vi "Scripted Autonmous V1.vi"(9 "All Autonmous Programs":T32, 10 "Autonmous Program":T1, 11 "Robot dev revs":T3={"Drive"={"Drive Actuaters"={"Motor devRevs"={"Left Side Motors"={"Motor 1 devRev"={"DeviceStatus"={"status"=FALSE, "code"=0, "source"=""}, "Type"=enum."PWM", "PWM"={"Digital Module"=enum."Digital Module 1", "PWM Channel"=enum."PWM 1", "DeadBand"={"Name"="", "maxPositivePwm"=0, "minPositivePwm"=0, "centerPwm"=0, "maxNegativePwm"=0, "minNegativePwm"=0, "angularRange"=0}}, "CAN"={"Device Number"=0, "Control Mode"=enum."Percent VBus", "Semaphore"=refnum, "Max Vout"=0.0}, "Invert"=FALSE, "TransformRef"=refnum, "InvTransformRef"=refnum}, "Motor 2 devRev"={"DeviceStatus"={"status"=FALSE, "code"=0, "source"=""}, "Type"=enum."PWM", "PWM"={"Digital Module"=enum."Digital Module 1", "PWM Channel"=enum."PWM 1", "DeadBand"={"Name"="", "maxPositivePwm"=0, "minPositivePwm"=0, "centerPwm"=0, "maxNegativePwm"=0, "minNegativePwm"=0, "angularRange"=0}}, "CAN"={"Device Number"=0, "Control Mode"=enum."Percent VBus", "Semaphore"=refnum, "Max Vout"=0.0}, "Invert"=FALSE, "TransformRef"=refnum, "InvTransformRef"=refnum}, "Motor 3 devRev"={"DeviceStatus"={"status"=FALSE, "code"=0, "source"=""}, "Type"=enum."PWM", "PWM"={"Digital Module"=enum."Digital Module 1", "PWM Channel"=enum."PWM 1", "DeadBand"={"Name"="", "maxPositivePwm"=0, "minPositivePwm"=0, "centerPwm"=0, "maxNegativePwm"=0, "minNegativePwm"=0, "angularRange"=0}}, "CAN"={"Device Number"=0, "Control Mode"=enum."Percent VBus", "Semaphore"=refnum, "Max Vout"=0.0}, "Invert"=FALSE, "TransformRef"=refnum, "InvTransformRef"=refnum}}, "Right Side Motors"={"Motor 1 devRev"={"DeviceStatus"={"status"=FALSE, "code"=0, "source"=""}, "Type"=enum."PWM", "PWM"={"Digital Module"=enum."Digital Module 1", "PWM Channel"=enum."PWM 1", "DeadBand"={"Name"="", "maxPositivePwm"=0, "minPositivePwm"=0, "centerPwm"=0, "maxNegativePwm"=0, "minNegativePwm"=0, "angularRange"=0}}, "CAN"={"Device Number"=0, "Control Mode"=enum."Percent VBus", "Semaphore"=refnum, "Max Vout"=0.0}, "Invert"=FALSE, "TransformRef"=refnum, "InvTransformRef"=refnum}, "Motor 2 devRev"={"DeviceStatus"={"status"=FALSE, "code"=0, "source"=""}, "Type"=enum."PWM", "PWM"={"Digital Module"=enum."Digital Module 1", "PWM Channel"=enum."PWM 1", "DeadBand"={"Name"="", "maxPositivePwm"=0, "minPositivePwm"=0, "centerPwm"=0, "maxNegativePwm"=0, "minNegativePwm"=0, "angularRange"=0}}, "CAN"={"Device Number"=0, "Control Mode"=enum."Percent VBus", "Semaphore"=refnum, "Max Vout"=0.0}, "Invert"=FALSE, "TransformRef"=refnum, "InvTransformRef"=refnum}, "Motor 3 devRev"={"DeviceStatus"={"status"=FALSE, "code"=0, "source"=""}, "Type"=enum."PWM", "PWM"={"Digital Module"=enum."Digital Module 1", "PWM Channel"=enum."PWM 1", "DeadBand"={"Name"="", "maxPositivePwm"=0, "minPositivePwm"=0, "centerPwm"=0, "maxNegativePwm"=0, "minNegativePwm"=0, "angularRange"=0}}, "CAN"={"Device Number"=0, "Control Mode"=enum."Percent VBus", "Semaphore"=refnum, "Max Vout"=0.0}, "Invert"=FALSE, "TransformRef"=refnum, "InvTransformRef"=refnum}}, "dev Status"={"status"=FALSE, "code"=0, "source"=""}}, "SolenoidDevRef"={"DevStatus"={"status"=FALSE, "code"=0, "source"=""}, "Solenoid Module"=enum."Solenoid Module 1", "Forward Solenoid Channel"=enum."Solenoid 1", "Reverse Solenoid Channel"=enum."Solenoid 1"}}, "Drive Sensor data"={"Encoders"={"Right Encoder"={"DevStatus"={"status"=FALSE, "code"=0, "source"=""}, "EncoderIndex"=enum."Enc 0", "CounterIndex"=enum."Ctr 0", "DistancePerCount"=0.0, "Decoding Type"=enum."1x"}}, "GyroDevRef"={"DevStatus"={"status"=FALSE, "code"=0, "source"=""}, "Analog Module"=enum."Analog Module 1", "Analog Channel"=enum."AI 1", "Offset"=0.0, "Gain (VoltsPerDegree/Second)"=0.0}, "Last commanded Angle"=0.0}}, "Catapult devrevs"={"MotorControlDeviceRef"={"DeviceStatus"={"status"=FALSE, "code"=0, "source"=""}, "Type"=enum."PWM", "PWM"={"Digital Module"=enum."Digital Module 1", "PWM Channel"=enum."PWM 1", "DeadBand"={"Name"="", "maxPositivePwm"=0, "minPositivePwm"=0, "centerPwm"=0, "maxNegativePwm"=0, "minNegativePwm"=0, "angularRange"=0}}, "CAN"={"Device Number"=0, "Control Mode"=enum."Percent VBus", "Semaphore"=refnum, "Max Vout"=0.0}, "Invert"=FALSE, "TransformRef"=refnum, "InvTransformRef"=refnum}, "SolenoidDevRef"={"DevStatus"={"status"=FALSE, "code"=0, "source"=""}, "Solenoid Module"=enum."Solenoid Module 1", "Forward Solenoid Channel"=enum."Solenoid 1", "Reverse Solenoid Channel"=enum."Solenoid 1"}, "first limit switch"={"DevStatus"={"status"=FALSE, "code"=0, "source"=""}, "DIO Channel"=enum."DIO 1", "Digital Module"=enum."Digital Module 1"}, "second limit switch"={"DevStatus"={"status"=FALSE, "code"=0, "source"=""}, "DIO Channel"=enum."DIO 1", "Digital Module"=enum."Digital Module 1"}}, "Drive Joystick"={"Device"=enum."USB 1"}, "Operator Joystick"={"Device"=enum."USB 1"}, "roller devrevs"={"SolenoidDevRef"={"DevStatus"={"status"=FALSE, "code"=0, "source"=""}, "Solenoid Module"=enum."Solenoid Module 1", "Forward Solenoid Channel"=enum."Solenoid 1", "Reverse Solenoid Channel"=enum."Solenoid 1"}, "MotorControlDeviceRef"={"DeviceStatus"={"status"=FALSE, "code"=0, "source"=""}, "Type"=enum."PWM", "PWM"={"Digital Module"=enum."Digital Module 1", "PWM Channel"=enum."PWM 1", "DeadBand"={"Name"="", "maxPositivePwm"=0, "minPositivePwm"=0, "centerPwm"=0, "maxNegativePwm"=0, "minNegativePwm"=0, "angularRange"=0}}, "CAN"={"Device Number"=0, "Control Mode"=enum."Percent VBus", "Semaphore"=refnum, "Max Vout"=0.0}, "Invert"=FALSE, "TransformRef"=refnum, "InvTransformRef"=refnum}, "DigitalInputDevRef"={"DevStatus"={"status"=FALSE, "code"=0, "source"=""}, "DIO Channel"=enum."Invalid", "Digital Module"=enum."Digital Module 1"}}, "Puncher devrevs"={"SolenoidDevRef"={"DevStatus"={"status"=FALSE, "code"=0, "source"=""}, "Solenoid Module"=enum."Solenoid Module 1", "Forward Solenoid Channel"=enum."Solenoid 1", "Reverse Solenoid Channel"=enum."Solenoid 1"}, "DigitalInputDevRef"={"DevStatus"={"status"=FALSE, "code"=0, "source"=""}, "DIO Channel"=enum."DIO 1", "Digital Module"=enum."Digital Module 1"}}}) -> (3 "Robot dev revs out":T3={"Drive"={"Drive Actuaters"={"Motor devRevs"={"Left Side Motors"={"Motor 1 devRev"={"DeviceStatus"={"status"=FALSE, "code"=0, "source"=""}, "Type"=enum."PWM", "PWM"={"Digital Module"=enum."Digital Module 1", "PWM Channel"=enum."PWM 1", "DeadBand"={"Name"="", "maxPositivePwm"=0, "minPositivePwm"=0, "centerPwm"=0, "maxNegativePwm"=0, "minNegativePwm"=0, "angularRange"=0}}, "CAN"={"Device Number"=0, "Control Mode"=enum."Percent VBus", "Semaphore"=refnum, "Max Vout"=0.0}, "Invert"=FALSE, "TransformRef"=refnum, "InvTransformRef"=refnum}, "Motor 2 devRev"={"DeviceStatus"={"status"=FALSE, "code"=0, "source"=""}, "Type"=enum."PWM", "PWM"={"Digital Module"=enum."Digital Module 1", "PWM Channel"=enum."PWM 1", "DeadBand"={"Name"="", "maxPositivePwm"=0, "minPositivePwm"=0, "centerPwm"=0, "maxNegativePwm"=0, "minNegativePwm"=0, "angularRange"=0}}, "CAN"={"Device Number"=0, "Control Mode"=enum."Percent VBus", "Semaphore"=refnum, "Max Vout"=0.0}, "Invert"=FALSE, "TransformRef"=refnum, "InvTransformRef"=refnum}, "Motor 3 devRev"={"DeviceStatus"={"status"=FALSE, "code"=0, "source"=""}, "Type"=enum."PWM", "PWM"={"Digital Module"=enum."Digital Module 1", "PWM Channel"=enum."PWM 1", "DeadBand"={"Name"="", "maxPositivePwm"=0, "minPositivePwm"=0, "centerPwm"=0, "maxNegativePwm"=0, "minNegativePwm"=0, "angularRange"=0}}, "CAN"={"Device Number"=0, "Control Mode"=enum."Percent VBus", "Semaphore"=refnum, "Max Vout"=0.0}, "Invert"=FALSE, "TransformRef"=refnum, "InvTransformRef"=refnum}}, "Right Side Motors"={"Motor 1 devRev"={"DeviceStatus"={"status"=FALSE, "code"=0, "source"=""}, "Type"=enum."PWM", "PWM"={"Digital Module"=enum."Digital Module 1", "PWM Channel"=enum."PWM 1", "DeadBand"={"Name"="", "maxPositivePwm"=0, "minPositivePwm"=0, "centerPwm"=0, "maxNegativePwm"=0, "minNegativePwm"=0, "angularRange"=0}}, "CAN"={"Device Number"=0, "Control Mode"=enum."Percent VBus", "Semaphore"=refnum, "Max Vout"=0.0}, "Invert"=FALSE, "TransformRef"=refnum, "InvTransformRef"=refnum}, "Motor 2 devRev"={"DeviceStatus"={"status"=FALSE, "code"=0, "source"=""}, "Type"=enum."PWM", "PWM"={"Digital Module"=enum."Digital Module 1", "PWM Channel"=enum."PWM 1", "DeadBand"={"Name"="", "maxPositivePwm"=0, "minPositivePwm"=0, "centerPwm"=0, "maxNegativePwm"=0, "minNegativePwm"=0, "angularRange"=0}}, "CAN"={"Device Number"=0, "Control Mode"=enum."Percent VBus", "Semaphore"=refnum, "Max Vout"=0.0}, "Invert"=FALSE, "TransformRef"=refnum, "InvTransformRef"=refnum}, "Motor 3 devRev"={"DeviceStatus"={"status"=FALSE, "code"=0, "source"=""}, "Type"=enum."PWM", "PWM"={"Digital Module"=enum."Digital Module 1", "PWM Channel"=enum."PWM 1", "DeadBand"={"Name"="", "maxPositivePwm"=0, "minPositivePwm"=0, "centerPwm"=0, "maxNegativePwm"=0, "minNegativePwm"=0, "angularRange"=0}}, "CAN"={"Device Number"=0, "Control Mode"=enum."Percent VBus", "Semaphore"=refnum, "Max Vout"=0.0}, "Invert"=FALSE, "TransformRef"=refnum, "InvTransformRef"=refnum}}, "dev Status"={"status"=FALSE, "code"=0, "source"=""}}, "SolenoidDevRef"={"DevStatus"={"status"=FALSE, "code"=0, "source"=""}, "Solenoid Module"=enum."Solenoid Module 1", "Forward Solenoid Channel"=enum."Solenoid 1", "Reverse Solenoid Channel"=enum."Solenoid 1"}}, "Drive Sensor data"={"Encoders"={"Right Encoder"={"DevStatus"={"status"=FALSE, "code"=0, "source"=""}, "EncoderIndex"=enum."Enc 0", "CounterIndex"=enum."Ctr 0", "DistancePerCount"=0.0, "Decoding Type"=enum."1x"}}, "GyroDevRef"={"DevStatus"={"status"=FALSE, "code"=0, "source"=""}, "Analog Module"=enum."Analog Module 1", "Analog Channel"=enum."AI 1", "Offset"=0.0, "Gain (VoltsPerDegree/Second)"=0.0}, "Last commanded Angle"=0.0}}, "Catapult devrevs"={"MotorControlDeviceRef"={"DeviceStatus"={"status"=FALSE, "code"=0, "source"=""}, "Type"=enum."PWM", "PWM"={"Digital Module"=enum."Digital Module 1", "PWM Channel"=enum."PWM 1", "DeadBand"={"Name"="", "maxPositivePwm"=0, "minPositivePwm"=0, "centerPwm"=0, "maxNegativePwm"=0, "minNegativePwm"=0, "angularRange"=0}}, "CAN"={"Device Number"=0, "Control Mode"=enum."Percent VBus", "Semaphore"=refnum, "Max Vout"=0.0}, "Invert"=FALSE, "TransformRef"=refnum, "InvTransformRef"=refnum}, "SolenoidDevRef"={"DevStatus"={"status"=FALSE, "code"=0, "source"=""}, "Solenoid Module"=enum."Solenoid Module 1", "Forward Solenoid Channel"=enum."Solenoid 1", "Reverse Solenoid Channel"=enum."Solenoid 1"}, "first limit switch"={"DevStatus"={"status"=FALSE, "code"=0, "source"=""}, "DIO Channel"=enum."DIO 1", "Digital Module"=enum."Digital Module 1"}, "second limit switch"={"DevStatus"={"status"=FALSE, "code"=0, "source"=""}, "DIO Channel"=enum."DIO 1", "Digital Module"=enum."Digital Module 1"}}, "Drive Joystick"={"Device"=enum."USB 1"}, "Operator Joystick"={"Device"=enum."USB 1"}, "roller devrevs"={"SolenoidDevRef"={"DevStatus"={"status"=FALSE, "code"=0, "source"=""}, "Solenoid Module"=enum."Solenoid Module 1", "Forward Solenoid Channel"=enum."Solenoid 1", "Reverse Solenoid Channel"=enum."Solenoid 1"}, "MotorControlDeviceRef"={"DeviceStatus"={"status"=FALSE, "code"=0, "source"=""}, "Type"=enum."PWM", "PWM"={"Digital Module"=enum."Digital Module 1", "PWM Channel"=enum."PWM 1", "DeadBand"={"Name"="", "maxPositivePwm"=0, "minPositivePwm"=0, "centerPwm"=0, "maxNegativePwm"=0, "minNegativePwm"=0, "angularRange"=0}}, "CAN"={"Device Number"=0, "Control Mode"=enum."Percent VBus", "Semaphore"=refnum, "Max Vout"=0.0}, "Invert"=FALSE, "TransformRef"=refnum, "InvTransformRef"=refnum}, "DigitalInputDevRef"={"DevStatus"={"status"=FALSE, "code"=0, "source"=""}, "DIO Channel"=enum."Invalid", "Digital Module"=enum."Digital Module 1"}}, "Puncher devrevs"={"SolenoidDevRef"={"DevStatus"={"status"=FALSE, "code"=0, "source"=""}, "Solenoid Module"=enum."Solenoid Module 1", "Forward Solenoid Channel"=enum."Solenoid 1", "Reverse Solenoid Channel"=enum."Solenoid 1"}, "DigitalInputDevRef"={"DevStatus"={"status"=FALSE, "code"=0, "source"=""}, "DIO Channel"=enum."DIO 1", "Digital Module"=enum."Digital Module 1"}}})   [LabVIEW 2013]
uses:
  Auto Text file code/All Autonmous Programs typedef.ctl
  Auto Text file code/Autonmous Program typedef.ctl
  Auto Text file code/Autonmous Scripting array typedef.ctl
  Robot dev revs.ctl
  Drive Code/Drive typedef.ctl
  Drive Code/Drive Motors Typedef.ctl
  Drive Code/GearBox Typedef.ctl
  <vilib>/Rock Robotics/WPI/MotorControl/WPI_MotorControlDeviceRef.ctl
  <vilib>/Rock Robotics/SystemInterfaces/Typedef/FPGA_TypedefDigitalModule.ctl
  <vilib>/Rock Robotics/SystemInterfaces/DIO/FPGA_DIOPWMChannel.ctl
  <vilib>/Rock Robotics/WPI/PWM/WPI_PWMDeadband.ctl
  <vilib>/Rock Robotics/WPI/CAN/Jaguar/SubVIs/WPI_CANJaguar_ControlMode.ctl
  <vilib>/Rock Robotics/WPI/PWM/WPI_PWMTransform_ConPane.ctl
  <vilib>/Rock Robotics/WPI/Solenoid/WPI_SolenoidDevRef.ctl
  <vilib>/Rock Robotics/SystemInterfaces/Typedef/FPGA_TypedefSolenoidModule.ctl
  <vilib>/Rock Robotics/WPI/Solenoid/WPI_SolenoidChannel.ctl
  Drive Code/Drive Sensor Typedef.ctl
  <vilib>/Rock Robotics/WPI/Encoder/WPI_EncoderDevRef.ctl
  <vilib>/Rock Robotics/SystemInterfaces/Encoder/FPGA_EncoderIdx.ctl
  <vilib>/Rock Robotics/SystemInterfaces/Counter/FPGA_CounterCtrSystemIndex.ctl
  <vilib>/Rock Robotics/WPI/Encoder/WPI_EncoderType.ctl
  <vilib>/Rock Robotics/WPI/Gyro/WPI_GyroDevRef.ctl
  <vilib>/Rock Robotics/SystemInterfaces/Typedef/FPGA_TypedefAnalogModule.ctl
  <vilib>/Rock Robotics/SystemInterfaces/AI/FPGA_AIChannel.ctl
  catapult code/catapult type def.ctl
  <vilib>/Rock Robotics/WPI/DigitalInput/WPI_DigitalInputDevRef.ctl
  <vilib>/Rock Robotics/SystemInterfaces/DIO/FPGA_DIOChannel.ctl
  <vilib>/Rock Robotics/WPI/Joystick/WPI_JoystickDevRef.ctl
  <vilib>/Rock Robotics/WPI/Joystick/WPI_JoystickDeviceEnum.ctl
  Roller V2/roller typedef.ctl
  Puncher/Puncher type.ctl
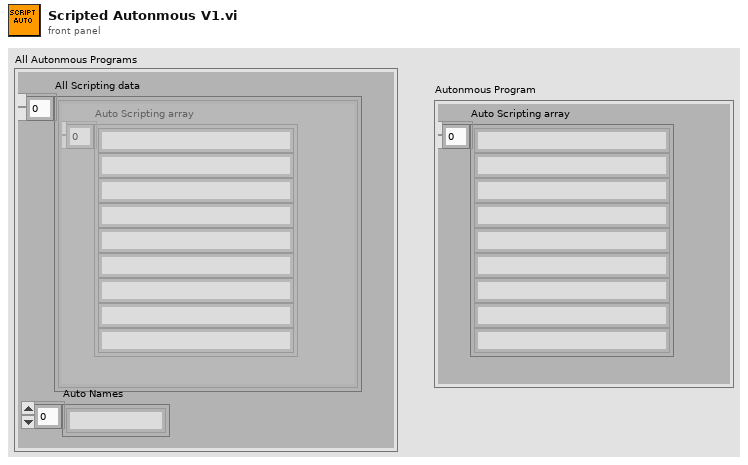
[diagram p1: front panel]
types:
  T1 = typedef "Autonmous Program typedef.ctl" = cluster{"Auto Scripting array":T2}
  T2 = typedef "Autonmous Scripting array typedef.ctl" = string[]
  T3 = typedef "Robot dev revs.ctl" = cluster{"Drive":T4, "Catapult devrevs":T25, "Drive Joystick":T28, "Operator Joystick":T28, "roller devrevs":T30, "Puncher devrevs":T31}
  T4 = typedef "Drive typedef.ctl" = cluster{"Drive Actuaters":cluster{"Motor devRevs":T5, "SolenoidDevRef":T14}, "Drive Sensor data":T17}
  T5 = typedef "Drive Motors Typedef.ctl" = cluster{"Left Side Motors":T6, "Right Side Motors":T6, "dev Status":errorcluster}
  T6 = typedef "GearBox Typedef.ctl" = cluster{"Motor 1 devRev":T7, "Motor 2 devRev":T7, "Motor 3 devRev":T7}
  T7 = typedef "WPI_MotorControlDeviceRef.ctl" = cluster{"DeviceStatus":errorcluster, "Type":enum16{"PWM", "CAN"}, "PWM":cluster{"Digital Module":T8, "PWM Channel":T9, "DeadBand":T10}, "CAN":cluster{"Device Number":u8, "Control Mode":T11, "Semaphore":T12, "Max Vout":dbl}, "Invert":bool, "TransformRef":T13, "InvTransformRef":T13}
  T8 = typedef "FPGA_TypedefDigitalModule.ctl" = enum16{"Digital Module 1", "Digital Module 2"}
  T9 = typedef "FPGA_DIOPWMChannel.ctl" = enum8{"PWM 1", "PWM 2", "PWM 3", "PWM 4", "PWM 5", "PWM 6", "PWM 7", "PWM 8", "PWM 9", "PWM 10", "Invalid"}
  T10 = typedef "WPI_PWMDeadband.ctl" = cluster{"Name":string, "maxPositivePwm":i32, "minPositivePwm":i32, "centerPwm":i32, "maxNegativePwm":i32, "minNegativePwm":i32, "angularRange":u16}
  T11 = typedef "WPI_CANJaguar_ControlMode.ctl" = enum8{"Percent VBus", "Current", "Speed", "Position", "Voltage"}
  T12 = typedef "Semaphore RefNum" = refnum<k1>
  T13 = typedef "WPI_PWMTransform_ConPane.ctl" = refnum<vi>
  T14 = typedef "WPI_SolenoidDevRef.ctl" = cluster{"DevStatus":errorcluster, "Solenoid Module":T15, "Forward Solenoid Channel":T16, "Reverse Solenoid Channel":T16}
  T15 = typedef "FPGA_TypedefSolenoidModule.ctl" = enum16{"Solenoid Module 1", "Solenoid Module 2"}
  T16 = typedef "WPI_SolenoidChannel.ctl" = enum8{"Solenoid 1", "Solenoid 2", "Solenoid 3", "Solenoid 4", "Solenoid 5", "Solenoid 6", "Solenoid 7", "Solenoid 8", "Invalid"}
  T17 = typedef "Drive Sensor Typedef.ctl" = cluster{"Encoders":cluster{"Right Encoder":T18}, "GyroDevRef":T22, "Last commanded Angle":dbl}
  T18 = typedef "WPI_EncoderDevRef.ctl" = cluster{"DevStatus":errorcluster, "EncoderIndex":T19, "CounterIndex":T20, "DistancePerCount":dbl, "Decoding Type":T21}
  T19 = typedef "FPGA_EncoderIdx.ctl" = enum8{"Enc 0", "Enc 1", "Enc 2", "Enc 3", "Invalid"}
  T20 = typedef "FPGA_CounterCtrSystemIndex.ctl" = enum8{"Ctr 0", "Ctr 1", "Ctr 2", "Ctr 3", "Ctr 4", "Ctr 5", "Ctr 6", "Ctr 7", "Invalid"}
  T21 = typedef "WPI_EncoderType.ctl" = enum16{"1x", "2x", "4x"}
  T22 = typedef "WPI_GyroDevRef.ctl" = cluster{"DevStatus":errorcluster, "Analog Module":T23, "Analog Channel":T24, "Offset":dbl, "Gain (VoltsPerDegree/Second)":dbl}
  T23 = typedef "FPGA_TypedefAnalogModule.ctl" = enum16{"Analog Module 1", "Analog Module 2"}
  T24 = typedef "FPGA_AIChannel.ctl" = enum8{"AI 1", "AI 2", "AI 3", "AI 4", "AI 5", "AI 6", "AI 7", "AI 8", "Invalid"}
  T25 = typedef "catapult type def.ctl" = cluster{"MotorControlDeviceRef":T7, "SolenoidDevRef":T14, "first limit switch":T26, "second limit switch":T26}
  T26 = typedef "WPI_DigitalInputDevRef.ctl" = cluster{"DevStatus":errorcluster, "DIO Channel":T27, "Digital Module":T8}
  T27 = typedef "FPGA_DIOChannel.ctl" = enum8{"DIO 1", "DIO 2", "DIO 3", "DIO 4", "DIO 5", "DIO 6", "DIO 7", "DIO 8", "DIO 9", "DIO 10", "DIO 11", "DIO 12", "DIO 13", "DIO 14", "Invalid"}
  T28 = typedef "WPI_JoystickDevRef.ctl" = cluster{"Device":T29}
  T29 = typedef "WPI_JoystickDeviceEnum.ctl" = enum16{"USB 1", "USB 2", "USB 3", "USB 4", "Kinect 1", "Kinect 2"}
  T30 = typedef "roller typedef.ctl" = cluster{"SolenoidDevRef":T14, "MotorControlDeviceRef":T7, "DigitalInputDevRef":T26}
  T31 = typedef "Puncher type.ctl" = cluster{"SolenoidDevRef":T14, "DigitalInputDevRef":T26}
  T32 = typedef "All Autonmous Programs typedef.ctl" = cluster{"All Scripting data":T1[], "Auto Names":string[]}
  T33 = cluster{"Forced high gear?":bool, "Force which gear it is in":bool}
  T34 = typedef "All Auto Drive constants.ctl" = cluster{"Drive auto Constants":T35, "All Shifter Constants":T36}
  T35 = typedef "Drive auto constants.ctl" = cluster{"PID Gains":cluster{"High Gear Gains":cluster{"PID Turn Gains":cluster{"proportional gain (Kc)":dbl, "integral time (Ti, min)":dbl, "derivative time (Td, min)":dbl}, "PID Straight Gains":cluster{"proportional gain (Kc)":dbl, "integral time (Ti, min)":dbl, "derivative time (Td, min)":dbl}}, "Low Gains":cluster{"PID Turn Gains":cluster{"proportional gain (Kc)":dbl, "integral time (Ti, min)":dbl, "derivative time (Td, min)":dbl}, "PID Straight Gains":cluster{"proportional gain (Kc)":dbl, "integral time (Ti, min)":dbl, "derivative time (Td, min)":dbl}}}, "Deadbands":cluster{"Turn Deadband":dbl, "Straight Deadband":dbl, "Mili seconds to wait to in deadband":u32}}
  T36 = typedef "All Shifter Constants.ctl" = cluster{"Drive info constants":cluster{"Enocder Pulses per foot":dbl, "Amount of turn before drive is turning":dbl}, "Shift control Constants":T37}
  T37 = typedef "Shift Constants.ctl" = cluster{"Global shift constants":cluster{"Mili seconds before it can shift again":u32, "Max fps":dbl}, "Upshift constants":cluster{"Upshift point in fps":dbl, "Upshift Accel constant":dbl, "Commanded Throttle  shiftpoint gain":dbl}, "Downshift Constants":cluster{"Kickdown shift point":dbl, "Kickdown at -acceleration":dbl, "Slowest Throttle for kickdown":dbl, "Coastdown shift speed":dbl}}
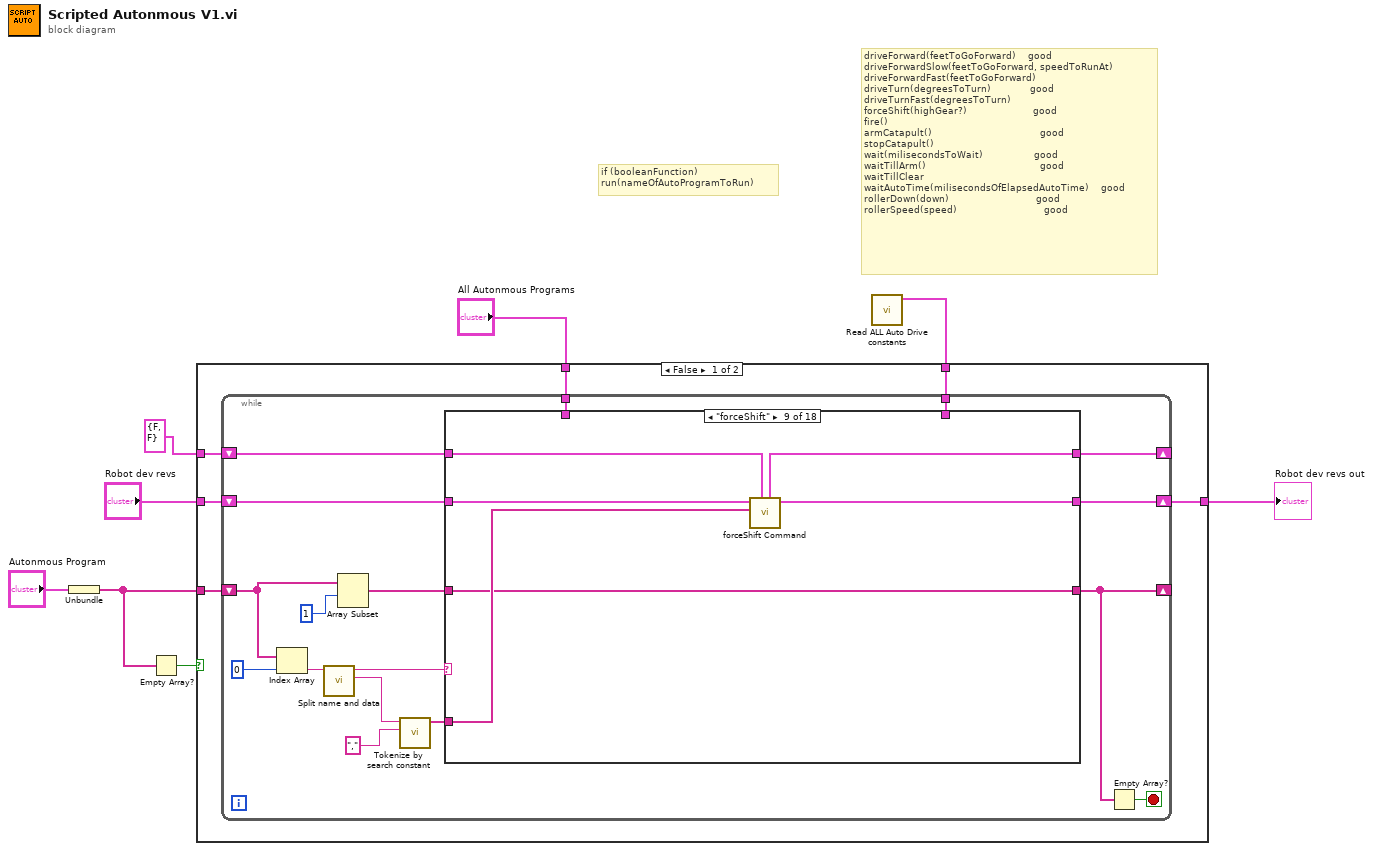
[diagram p0: block diagram]
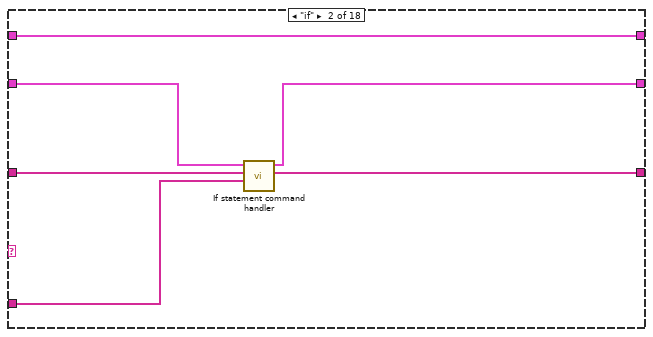
[diagram p3: hidden frame]
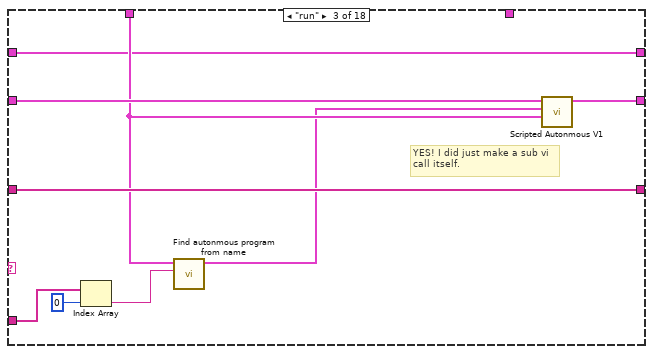
[diagram p4: hidden frame]
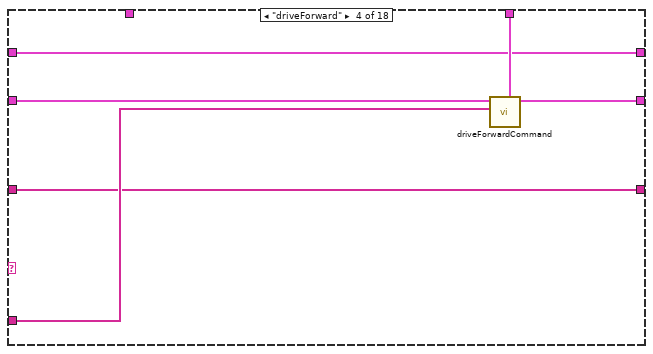
[diagram p5: hidden frame]
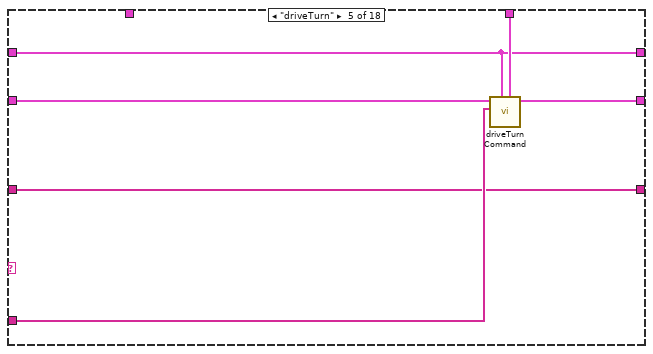
[diagram p6: hidden frame]
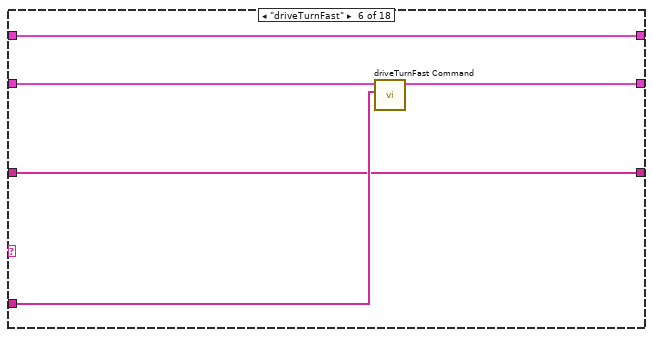
[diagram p7: hidden frame]
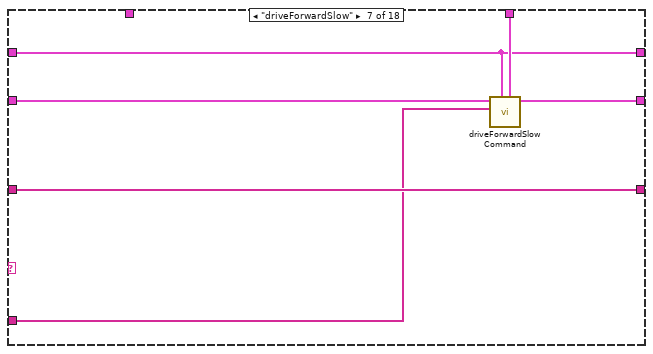
[diagram p8: hidden frame]
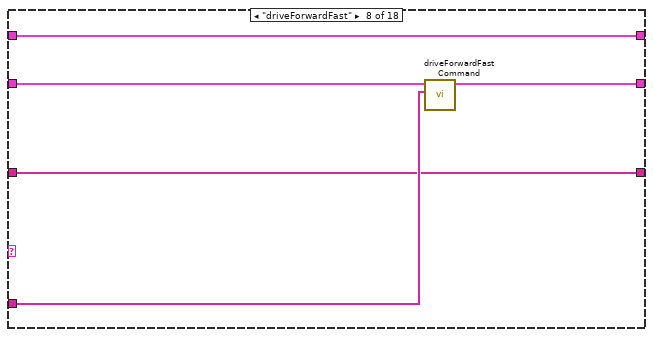
[diagram p9: hidden frame]
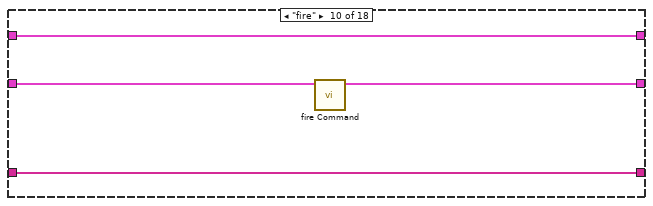
[diagram p10: hidden frame]
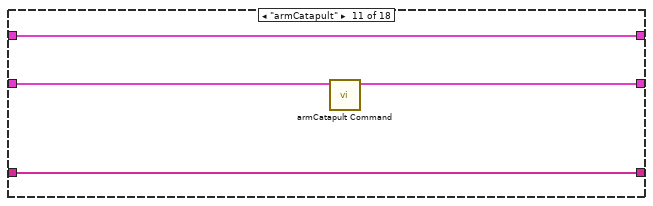
[diagram p11: hidden frame]
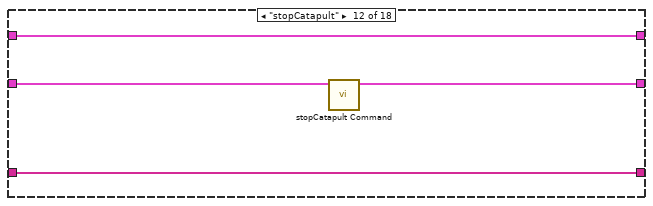
[diagram p12: hidden frame]
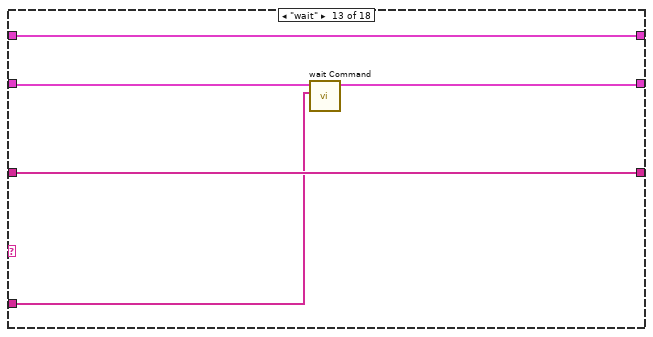
[diagram p13: hidden frame]
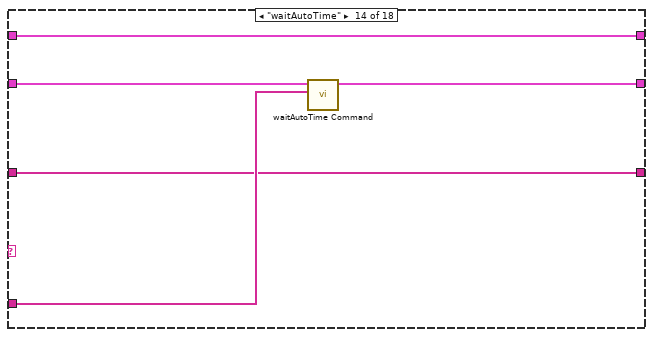
[diagram p14: hidden frame]
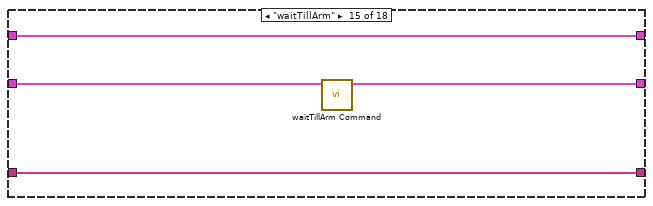
[diagram p15: hidden frame]
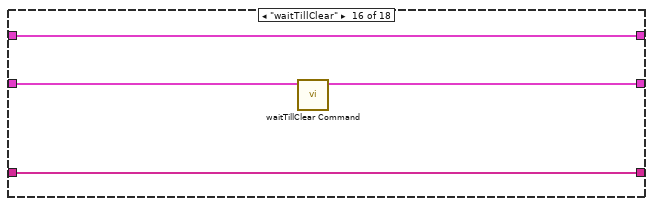
[diagram p16: hidden frame]
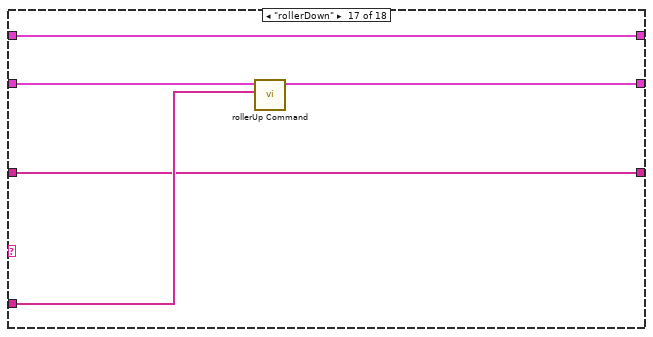
[diagram p17: hidden frame]
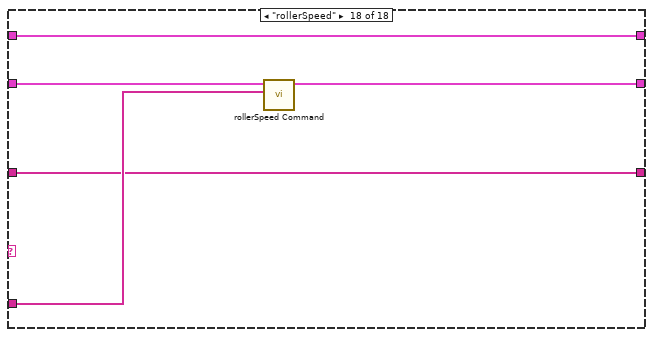
[diagram p18: hidden frame]
diagram:
  # "if (booleanFunction)\nrun(nameOfAutoProgramToRun)"
  # "driveForward(feetToGoForward)    good\ndriveForwardSlow(feetToGoForward, speedToRunAt)\ndriveForwardFast(feetToGoForward)\ndriveTurn(degreesToTurn)             good\ndriveTurnFast(degreesToTurn)\nforceShift(highGear?)                      good\nfire()\narmCatapult()                                    good\nstopCatapult()\nwait(milisecondsToWait)                 good\nwaitTillArm()                                      good\nwaitTillClear\nwaitAutoTime(milisecondsOfElapsedAutoTime)    good\nrollerDown(down)                             good\nrollerSpeed(speed)                             good"
  n1 = Unbundle("Autonmous Program") -> ("Auto Scripting array"=w3:T2)
  n2 = Empty Array?(array=w3) -> (empty?=w5:bool)
  n3 = call "Read ALL Auto Drive constants.vi"() -> ("All Drive Constants"=w2:T34)  [unwired: 10 in, 1 out]
  n4 = case shown="False" w5 {
    tunnel: "All Autonmous Programs" -> [w14 _]
    tunnel: "Robot dev revs" -> [w13 w124]
    tunnel: [w12 w124] -> w6
    tunnel: w3 -> [w11 _]
    tunnel: w2 -> [w10 _]
    tunnel: T33 {"Forced high gear?"=FALSE, "Force which gear it is in"=FALSE} ("Shifting controls") -> [w9 _]
    frame False {
      n5 = while {
        shift-right: [w22] -> _
        shift-left: w11 -> [w24]
        tunnel: w14 -> [w21]
        shift-right: [w19] -> w12
        shift-left: w13 -> [w20]
        tunnel: w10 -> [w17]
        shift-right: [w15] -> _
        shift-left: w9 -> [w16]
        stop <- w27 stop-if-true
        n6 = Index Array(array=w24, index=0) -> (element=w28:string)
        n7 = call "Split name and data.vi"("string"=w28) -> ("Data"=w30:string, "Command Name"=w31:string)  [unwired: 9 in]
        n8 = Array Subset(array=w24, index=1) -> (w23:T2)  [unwired: 1 in]
        n9 = call "Tokenize by search constant.vi"("search constant"=",", "Data"=w30) -> ("Array"=w29:string[])  [unwired: 9 in]
        n10 = case shown="\"forceShift\"" w31 {
          tunnel: w29 -> [_ w40 w46 w54 w58 w64 w68 w74 w79 _ _ _ w98 w103 _ _ w116 w121]
          tunnel: w23 -> [w34 w39 w49 w53 w57 w63 w69 w73 w78 w84 w89 w92 w100 w101 w107 w110 w115 w120]
          tunnel: [w34 w38 w49 w53 w57 w63 w69 w73 w78 w84 w89 w92 w100 w101 w107 w110 w115 w120] -> w22
          tunnel: w21 -> [_ _ w43 _ _ _ _ _ _ _ _ _ _ _ _ _ _ _]
          tunnel: w20 -> [w33 w37 w48 w55 w60 w66 w72 w77 w83 w87 w91 w95 w99 w105 w109 w113 w118 w123]
          tunnel: [w33 w36 w47 w52 w61 w65 w70 w76 w82 w86 w90 w94 w97 w104 w108 w112 w117 w122] -> w19
          tunnel: w17 -> [_ _ _ w51 w59 _ w71 _ _ _ _ _ _ _ _ _ _ _]
          tunnel: [w32 w35 w41 w50 w56 w62 w67 w75 w81 w85 w88 w93 w96 w102 w106 w111 w114 w119] -> w15
          tunnel: w16 -> [w32 w35 w41 w50 w56 w62 w67 w75 w80 w85 w88 w93 w96 w102 w106 w111 w114 w119]
          frame "", Default {
          }
          frame "if" {
            n11 = call "If statement command handler.vi"("Data"=w40, "Auto Scripting array"=w39, "Robot dev revs"=w37) -> ("Auto Scripting array out"=w38:T2, "Robot dev revs out"=w36:T3)  [unwired: 7 in]
          }
          frame "run" {
            # "YES! I did just make a sub vi\ncall itself."
            n12 = Index Array(array=w46, index=0) -> (element=w44:string)
            n13 = call "Find autonmous program from name.vi"("Program Name"=w44, "All Autonmous Programs"=w43) -> ("Autonmous Program"=w42:T1)  [unwired: 8 in, 1 out]
            n14 = call "Scripted Autonmous V1.vi"("All Autonmous Programs"=w43, "Autonmous Program"=w42, "Robot dev revs"=w48) -> ("Robot dev revs out"=w47:T3)  [unwired: 8 in]
          }
          frame "driveForward" {
            n15 = call "driveForwardCommand.vi"("All Auto Drive constants"=w51, "Data"=w54, "Robot dev revs"=w55) -> ("Robot dev revs"=w52:T3)  [unwired: 8 in]
          }
          frame "driveTurn" {
            n16 = call "driveTurn Command.vi"("All Auto Drive constants"=w59, "Shifting controls"=w56, "Data"=w58, "Robot dev revs"=w60) -> ("Robot dev revs out"=w61:T3)  [unwired: 7 in]
          }
          frame "driveTurnFast" {
            n17 = call "driveTurnFast Command.vi"("Data"=w64, "Robot dev revs"=w66) -> ("Robot dev revs out"=w65:T3)  [unwired: 9 in]
          }
          frame "driveForwardSlow" {
            n18 = call "driveForwardSlow Command.vi"("All Auto Drive constants"=w71, "Shifting controls"=w67, "Data"=w68, "Robot dev revs"=w72) -> ("Robot dev revs out"=w70:T3)  [unwired: 7 in]
          }
          frame "driveForwardFast" {
            n19 = call "driveForwardFast Command.vi"("Data"=w74, "Robot dev revs"=w77) -> ("Robot dev revs out"=w76:T3)  [unwired: 9 in]
          }
          frame "forceShift" {
            n20 = call "forceShift Command.vi"("Shifting controls"=w80, "Data"=w79, "Robot dev revs"=w83) -> ("Robot dev revs out"=w82:T3, "Shifting controls out"=w81:T33)  [unwired: 7 in]
          }
          frame "fire" {
            n21 = call "fire Command.vi"("Robot dev revs"=w87) -> ("Robot dev revs out"=w86:T3)  [unwired: 10 in]
          }
          frame "armCatapult" {
            n22 = call "armCatapult Command.vi"("Robot dev revs"=w91) -> ("Robot dev revs out"=w90:T3)  [unwired: 10 in]
          }
          frame "stopCatapult" {
            n23 = call "stopCatapult Command.vi"("Robot dev revs in"=w95) -> ("Robot dev revs out"=w94:T3)  [unwired: 10 in]
          }
          frame "wait" {
            n24 = call "wait Command.vi"("Data"=w98, "Robot dev revs"=w99) -> ("Robot dev revs 2"=w97:T3)  [unwired: 9 in]
          }
          frame "waitAutoTime" {
            n25 = call "waitAutoTime Command.vi"("Array"=w103, "Robot dev revs in"=w105) -> ("Robot dev revs out"=w104:T3)  [unwired: 9 in]
          }
          frame "waitTillArm" {
            n26 = call "waitTillArm Command.vi"("Robot dev revs in"=w109) -> ("Robot dev revs out"=w108:T3)  [unwired: 10 in]
          }
          frame "waitTillClear" {
            n27 = call "waitTillClear Command.vi"("Robot dev revs in"=w113) -> ("Robot dev revs out"=w112:T3)  [unwired: 10 in]
          }
          frame "rollerDown" {
            n28 = call "rollerUp Command.vi"("Data"=w116, "Robot dev revs"=w118) -> ("Robot dev revs out"=w117:T3)  [unwired: 9 in]
          }
          frame "rollerSpeed" {
            n29 = call "rollerSpeed Command.vi"("Data"=w121, "Robot dev revs"=w123) -> ("Robot dev revs out"=w122:T3)  [unwired: 9 in]
          }
        }
        n30 = Empty Array?(array=w22) -> (empty?=w27:bool)
      }
    }
    frame True {
      # "Don't do anything if the scripting is empty"
    }
  }
  "Robot dev revs out" <- w6
